vi "unterbrechbares_wait.vi"() -> ()   [LabVIEW 2013]
uses:
  global_notaus.vi
panel:
  in  "Notaus":bool
  in  "max. wait time":u32=2000
  in  "Wait":bool
  in  "Stopp":bool
  out "Aktuelle Zeit":timestamp
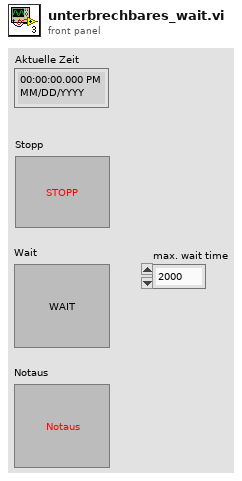
[diagram p1: front panel]
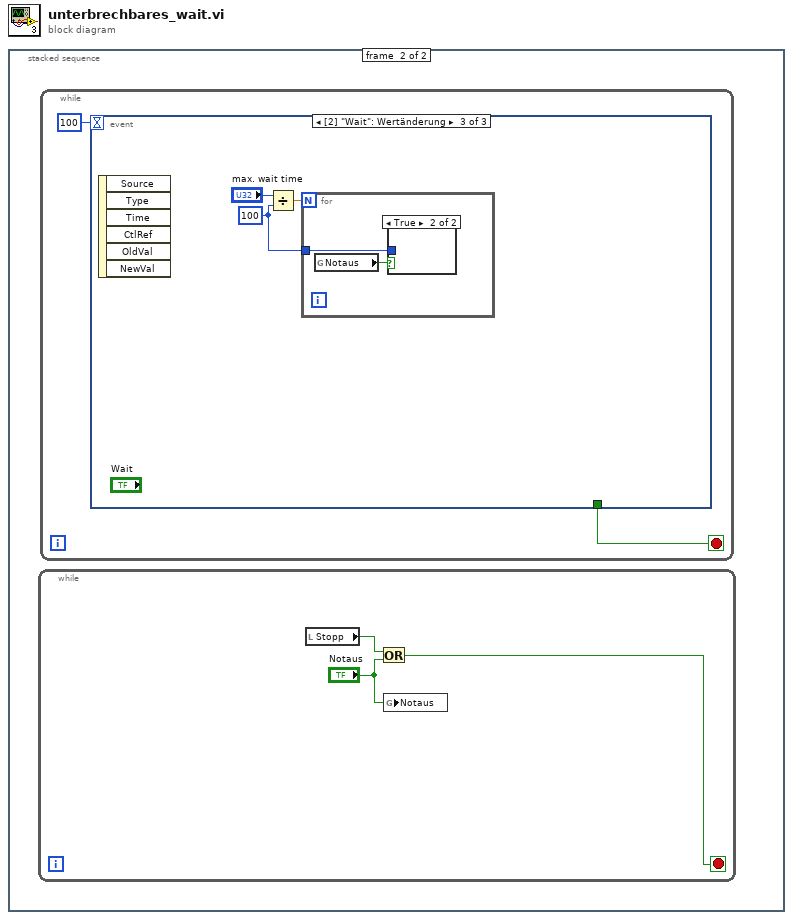
[diagram p0: block diagram]
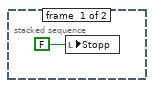
[diagram p2: hidden frame]
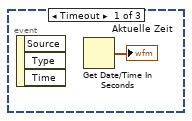
[diagram p3: hidden frame]
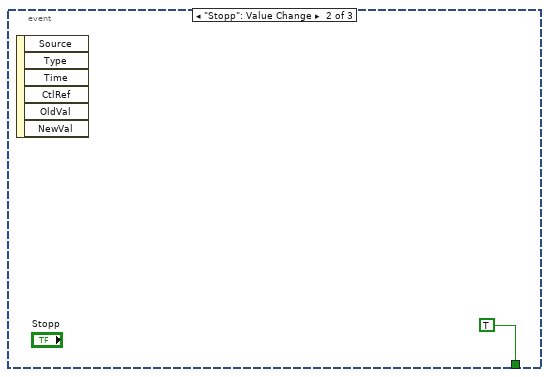
[diagram p4: hidden frame]
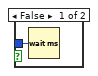
[diagram p5: hidden frame]
diagram:
  n1 = stacked-sequence {
    frame #0 {
      n2 = local write "Stopp"(FALSE) -> ()
    }
    frame #1 {
      n3 = while {
        stop <- w3 stop-if-true
        n4 = local read "Stopp"() -> (w4:bool)
        n5 = Or(x=w4, y="Notaus") -> (x .or. y?=w3:bool)
        n6 = global write "global_notaus.vi" "Notaus"("Notaus") -> ()
      }
      n7 = while {
        stop <- w5 stop-if-true
        n8 = event shown="[2] \"Wait\": Wertänderung" {
          selector: _ -> [_ _ _]
          dyn-events: _ -> [_ _ _]
          timeout: 100 -> [_ _ _]
          tunnel: [_ TRUE _] -> w5
          event Timeout {
            n9 = event-data() -> ()  [unwired: 1 in, 3 out]
            n10 = Get Date/Time In Seconds() -> (seconds since 1Jan1904=→"Aktuelle Zeit":timestamp)
          }
          event "Stopp": Value Change {
            n11 = event-data() -> ()  [unwired: 1 in, 6 out]
          }
          event "Wait": Value Change {
            w9 = u32 100 ("y")
            n12 = event-data() -> ()  [unwired: 1 in, 6 out]
            n13 = Divide(x="max. wait time", y=w9) -> (x/y=w10:dbl)
            n14 = for {
              N: w10 -> [_]
              tunnel: w9 -> [w13]
              n15 = global read "global_notaus.vi" "Notaus"() -> (w12:bool)
              n16 = case shown="True" w12 {
                tunnel: w13 -> [w14 _]
                frame False {
                  n17 = Wait (ms)(milliseconds to wait=w14) -> ()  [unwired: 1 out]
                }
                frame True {
                }
              }
            }
          }
        }
      }
    }
  }
